vi "Application Data.vi"() -> ()   [LabVIEW 2014]
uses:
  Track Controls.ctl
  Track Volume Settings.ctl
  Sub VIs/Audio/Controls/playback state.ctl
panel:
  in  "Delay":u32
  in  "Track Name":string
  in  "Frequency":dbl
  in  "stop":bool
  in  "Playback State":T1=enum."Play"
  in  "Track Controls":T2 {"Track 3"."Volume" scale=0.01..10.0; "Track 3"."Pan" scale=0.0..1.0; "Track 2"."Volume" scale=0.01..10.0; "Track 2"."Pan" scale=0.0..1.0; "Track 1"."Volume" scale=0.01..10.0; "Track 1"."Pan" scale=0.0..1.0; "Track 0"."Volume" scale=0.01..10.0; "Track 0"."Pan" scale=0.0..1.0}
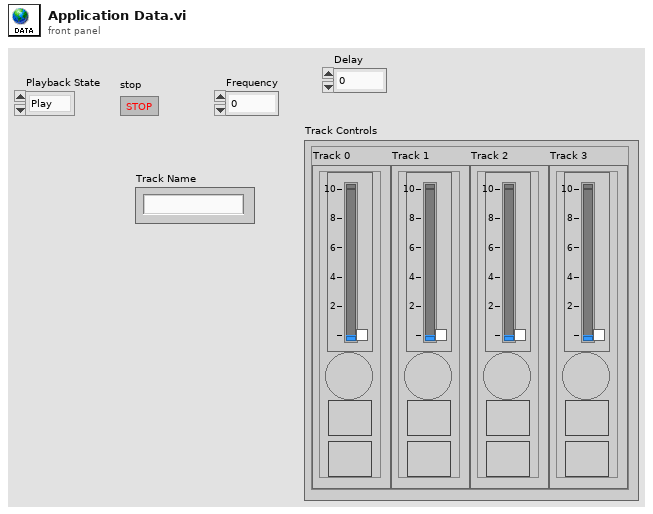
[diagram p1: front panel]
types:
  T1 = typedef "playback state.ctl" = enum16{"Load File", "Save File", "Play", "Record", "Stop", "Rewind"}
  T2 = typedef "Track Controls.ctl" = cluster{"Track 0":T3, "Track 1":T3, "Track 2":T3, "Track 3":T3}
  T3 = typedef "Track Volume Settings.ctl" = cluster{"Volume":dbl, "Pan":dbl, "Record":bool, "FX":bool}
diagram:
